vi "ROS_Topic_Reply.vi"(0 "data":T4={"New Subscriber"={"Caller ID"="", "Topic Name"="", "Protocol"="", "URIs"="", "ID"=refnum}, "ROS of Server"={"topic port"=0, "Node"="", "topic"="", "type"="", "node port"=0, "error "={"status"=FALSE, "code"=0, "source"=""}, "Direction"=enum."Node", "APIs"=[], "Update (ms)"=1, "write queue"=1}, "new port"=0}, 1 "My ROS":T1={"topic port"=1236, "Node"="/labview", "topic"="/robot/head/command_head_nod", "type"="std_msgs/Bool", "node port"=7000, "error "={"status"=FALSE, "code"=0, "source"=""}, "Direction"=enum."Publisher", "APIs"=[], "Update (ms)"=1, "write queue"=1}) -> (2 "Subscriber out":T3, 3 "Log":T5, 4 "error IO":errorcluster)   [LabVIEW 2012]
uses:
  Console/Servers/ServerSubs/ROSLog.ctl
  Console/Servers/ServerSubs/MyState.ctl
  _ROSDefinition.vi
  SubVIs/_ROSDirection.ctl
  SubVIs/_ROSControl.ctl
  Console/Servers/ServerSubs/requestTopic.ctl
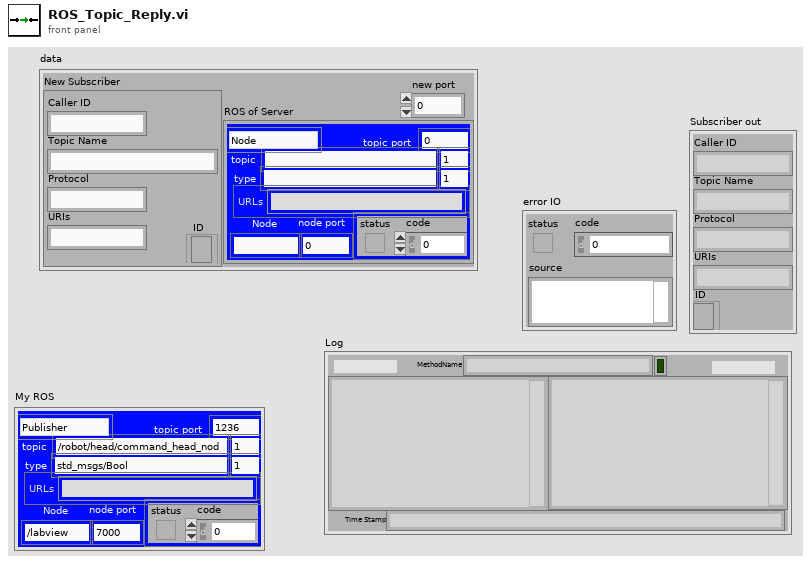
[diagram p1: front panel]
types:
  T1 = typedef "_ROSControl.ctl" = cluster{"topic port":u16, "Node":string, "topic":string, "type":string, "node port":u32, "error ":errorcluster, "Direction":T2, "APIs":string[], "Update (ms)":u16, "write queue":u16}
  T2 = typedef "_ROSDirection.ctl" = enum16{"Node", "Publisher", "Subscriber", "Service Client"}
  T3 = cluster{"Caller ID":string, "Topic Name":string, "Protocol":string, "URIs":string, "ID":refnum<k5>}
  T4 = typedef "requestTopic.ctl" = cluster{"New Subscriber":cluster{"Caller ID":string, "Topic Name":string, "Protocol":string, "URIs":string, "ID":refnum<k5>}, "ROS of Server":T1, "new port":u16}
  T5 = typedef "ROSLog.ctl" = cluster{"Sent":string, "Reply":string, "MethodName":string, "success":bool, "Dir1":string, "Dir2":string, "Time Stamp":string}
  T6 = typedef "MyState.ctl" = enum16{"No Connection", "Registered", "Connected", "Close"}
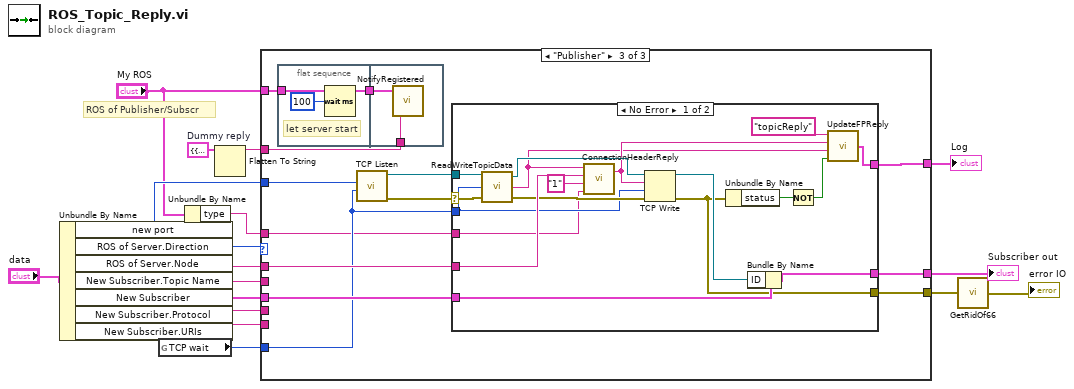
[diagram p0: block diagram]
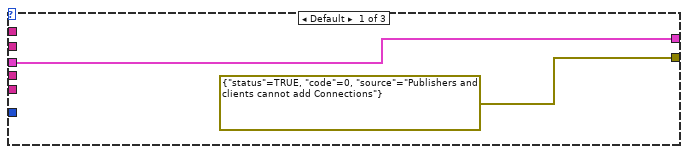
[diagram p2: hidden frame]
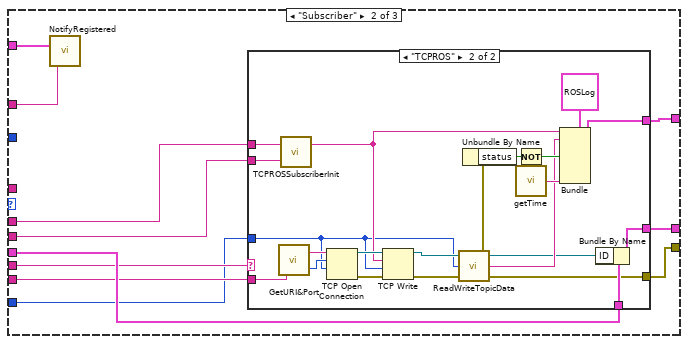
[diagram p3: hidden frame]
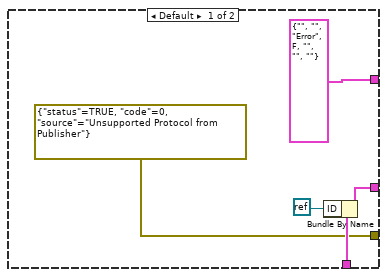
[diagram p4: hidden frame]
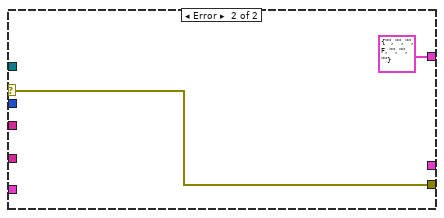
[diagram p5: hidden frame]
diagram:
  w6 = cluster{"Log":T5, "MyState":T6} {"Log"={"Sent"="Dummy notify for req topic", "Reply"="", "MethodName"="", "success"=FALSE, "Dir1"="", "Dir2"="", "Time Stamp"=""}, "MyState"=enum."Registered"}  # Dummy reply
  # "ROS of Publisher/Subscr"
  n1 = Unbundle By Name("data") -> ("new port"=w14:u16, "ROS of Server.Direction"=w10:T2, "ROS of Server.Node"=w16:string, "New Subscriber.Topic Name"=w17:string, "New Subscriber"=w13:T3, "New Subscriber.Protocol"=w8:string, "New Subscriber.URIs"=w9:string)
  n2 = global read "_ROSDefinition.vi" "TCP wait"() -> (w7:i32)
  n3 = Unbundle By Name("My ROS") -> ("type"=w3:string)
  n4 = Flatten To String(anything=w6) -> (data string=w5:string)  [unwired: 3 in, 2 out]
  n5 = case shown="\"Publisher\"" w10 {
    tunnel: w17 -> [_ w28 _]
    tunnel: w16 -> [_ w29 w67]
    tunnel: [w19 w26 w66] -> w15
    tunnel: [errorcluster {"status"=TRUE, "code"=0, "source"="Publishers and clients cannot add Connections"} ("error IO") w25 w65] -> w2
    tunnel: w14 -> [_ _ w64]
    tunnel: w13 -> [w19 w27 w63]
    tunnel: [_ w30 w62] -> w11
    tunnel: w9 -> [_ w23 _]
    tunnel: w8 -> [_ w24 _]
    tunnel: "My ROS" -> [_ w21 w61]
    tunnel: w7 -> [_ w22 w60]
    tunnel: w5 -> [_ w20 w58]
    tunnel: w3 -> [_ _ w57]
    frame Default {
    }
    frame "Subscriber" {
      n6 = call "NotifyRegistered.vi"("data string"=w20, "ROS"=w21) -> ()  [unwired: 2 in]
      n7 = case shown="\"TCPROS\"" w24 {
        tunnel: [T5 {"Sent"="", "Reply"="", "MethodName"="Error", "success"=FALSE, "Dir1"="", "Dir2"="", "Time Stamp"=""} ("Log") w46] -> w30
        tunnel: w29 -> [_ w45]
        tunnel: w28 -> [_ w44]
        tunnel: w27 -> [w35 w41]
        tunnel: [w33 w40] -> w26
        tunnel: [errorcluster {"status"=TRUE, "code"=0, "source"="Unsupported Protocol from Publisher"} ("error out") w38] -> w25
        tunnel: w23 -> [_ w37]
        tunnel: w22 -> [_ w36]
        frame Default {
          n8 = Bundle By Name(cluster=w35, "ID"=refnum<k0> refnum) -> (w33:T3)
        }
        frame "TCPROS" {
          n9 = call "GetURI&Port.vi"("URI in"=w37) -> ("Port"=w55:u16, "URI"=w56:string)
          n10 = call "TCPROSSubscriberInit.vi"("topic"=w44, "callerID"=w45) -> ("TCP ROS Reply"=w43:string)  [unwired: 1 in]
          n11 = TCP Open Connection(address=w56, remote port or service name=w55, timeout ms (60000)=w36) -> (connection ID=w54:refnum<k5>, error out=w53:errorcluster)  [unwired: 2 in]
          n12 = TCP Write(connection ID=w54, data in=w43, error in (no error)=w53, 9:w36) -> (connection ID out=w52:refnum<k5>, error out=w51:errorcluster)  [unwired: 1 out]
          n13 = call "ReadWriteTopicData.vi"("error in (no error)"=w51, "timeout ms (1000)"=w36, "connection ID in"=w52) -> ("error out"=w38:errorcluster, "data out"=w42:string, "connection ID out"=w39:refnum<k5>)
          n14 = Unbundle By Name(w38) -> ("status"=w49:bool)
          n15 = Not(x=w49) -> (.not. x?=w48:bool)
          n16 = call "getTime.vi"() -> ("Current Time"=w47:string)  [unwired: 1 in]
          n17 = Bundle(cluster=T5 {"Sent"="", "Reply"="", "MethodName"="Publisher ID", "success"=FALSE, "Dir1"="To ROS", "Dir2"="From ROS", "Time Stamp"=""} ("Log"), "Sent"=w43, "Reply"=w42, "success"=w48, "Time Stamp"=w47) -> (w46:T5)  [unwired: 3 in]
          n18 = Bundle By Name(cluster=w41, "ID"=w39) -> (w40:T3)
        }
      }
    }
    frame "Publisher" {
      n19 = flat-sequence {
        tunnel: w61 -> [w71]
        tunnel: [w71] -> w59
        tunnel: w59 -> [w73]
        tunnel: w58 -> [w72]
        frame #0 {
          # "let server start"
          n20 = Wait (ms)(milliseconds to wait=u32 100) -> ()  [unwired: 1 out]
        }
        frame #1 {
          n21 = call "NotifyRegistered.vi"("data string"=w72, "ROS"=w73) -> ()  [unwired: 2 in]
        }
      }
      n22 = call <vilib>:"TCP Listen.vi"("timeout ms (wait forever: -1)"=w60, "port"=w64) -> ("error out"=w69:errorcluster, "connection ID"=w68:refnum<k5>)  [unwired: 5 in, 3 out]
      n23 = case shown="No Error" w69 {
        selector: w69 -> [w90 w93]
        tunnel: w68 -> [w91 _]
        tunnel: w67 -> [w89 _]
        tunnel: [w74 w93] -> w65
        tunnel: w63 -> [w80 _]
        tunnel: [w78 _] -> w66
        tunnel: [w81 T5 {"Sent"="", "Reply"="", "MethodName"="", "success"=FALSE, "Dir1"="", "Dir2"="", "Time Stamp"=""} ("Log")] -> w62
        tunnel: w60 -> [w76 _]
        tunnel: w57 -> [w75 _]
        frame No Error {
          n24 = call "ReadWriteTopicData.vi"("error in (no error)"=w90, "timeout ms (1000)"=w76, "connection ID in"=w91) -> ("error out"=w86:errorcluster, "data out"=w84:string, "connection ID out"=w87:refnum<k5>)
          n25 = call "ConnectionHeaderReply.vi"("type"=w75, "Latching"="1", "Caller ID"=w89, "TCPROS Connection Header"=w84) -> ("Connection Response"=w85:string)  [unwired: 1 in]
          n26 = TCP Write(connection ID=w87, data in=w85, error in (no error)=w86, 9:w76) -> (connection ID out=w79:refnum<k5>, error out=w74:errorcluster)  [unwired: 1 out]
          n27 = Unbundle By Name(w74) -> ("status"=w77:bool)
          n28 = Bundle By Name(cluster=w80, "ID"=w79) -> (w78:T3)
          n29 = Not(x=w77) -> (.not. x?=w83:bool)
          n30 = call "UpdateFPReply.vi"("success?"=w83, "Reply"=w84, "Sent"=w85, "method"="topicReply") -> ("Log"=w81:T5)
        }
        frame Error {
        }
      }
    }
  }
  "Log" <- w11
  "Subscriber out" <- w15
  n31 = call "GetRidOf66.vi"("error in (no error)"=w2) -> ("error out"=→"error IO":errorcluster)
